vi "Dashboard Main.vi"() -> ()   [LabVIEW 2014]
uses:
  AutonModes.ctl
  <vilib>/event_ctls.llb/eventvkey.ctl
  <vilib>/Rock Robotics/WPI/Dashboard/WPI_DashboardLogging Global.vi
  <vilib>/Rock Robotics/Network Tables/SD Write String.vi
  <vilib>/Utility/config.llb/Write Key (String).vi
  <vilib>/Utility/config.llb/Write Key (I32).vi
  <vilib>/Utility/config.llb/NI_LVConfig.lvlib
panel:
  in  "TCP":refnum<k5>
  in  "Rec Mode":enum32{"Stop", "Record", "Playback"}(radio)
  in  "Vision":u16(ring) items=["Camera Off", "USB Camera SW", "USB Camera HW", "IP Camera"]
  out "Camera IP":string
  out "Image Message":string="Timeout in Camera Communications"
  in  "Dashboard Tab":T1(tab)
  in  "Camera Settings":T2={"Frame Rate"=30, "Compression"=30, "Size"=1} {"Frame Rate" scale=1.0..30.0; "Size" items=["640x480", "320x240", "160x120"]}
  out "MotorChart R":cluster{"Numeric":dbl, "Numeric":dbl}(graph)
  out "MotorChart L":T3(graph)
  out "MotorSliders R":cluster{"MotorSlide1":dbl, "MotorSlide2":dbl} {"MotorSlide2" scale=-1.0..1.0 scale format="%#_2e"; "MotorSlide1" scale=-1.0..1.0 scale format="%#_2e"}
  out "MotorSliders L":T4 {"MotorSlide4 2" scale=0.0..14.0 scale format="%#_2e"; "MotorSlide2" scale=-1.0..1.0 scale format="%#_2e"; "MotorSlide1" scale=-1.0..1.0 scale format="%#_2e"}
  out "Gyro":dbl(knob) scale=0.0..360.0
  out "JS1 Z":dbl(slide) scale=-1.0..1.0 scale format="%#_2e"
  out "JS1 Graph":cluster{"X":dbl, "Y":dbl}[](graph)
  out "JS1 Buttons":T5
  out "JS2 Z":dbl(slide) scale=-1.0..1.0 scale format="%#_2e"
  out "JS2 Graph":cluster{"X":dbl, "Y":dbl}[](graph)
  out "JS2 Buttons":T5
  out "Mode":T6(ring)=enum."Auto Disabled"
  in  "DB Camera Config":bool
  out "fps":dbl format="%#.1g"
  out "Mbps":dbl format="%#.1g"
  out "Mbps 2":bool
  in  "Auton Mode":T7
  in  "DB/String 9":string
  in  "DB/String 8":string
  in  "DB/String 7":string
  in  "DB/String 6":string
  in  "DB/String 5":string
  in  "DB/String 4":string
  in  "DB/String 3":string
  in  "DB/String 2":string
  in  "DB/String 1":string
  in  "DB/String 0":string
  in  "DB/Slider 0":dbl(slide) scale=0.0..5.0
  in  "DB/Slider 1":dbl(slide) scale=0.0..5.0
  in  "DB/Slider 2":dbl(slide) scale=0.0..5.0
  in  "DB/Slider 3":dbl(slide) scale=0.0..5.0
  out "DB/LED 3":bool
  out "DB/LED 2":bool
  out "DB/LED 1":bool
  out "DB/LED 0":bool
  in  "DB/Button 3":bool
  in  "DB/Button 2":bool
  in  "DB/Button 1":bool
  in  "DB/Button 0":bool caption="New Name"
  in  "Test Slider":dbl(slide) scale=0.0..100.0 scale format="%#_3g"
  in  "On/Off":bool caption="Solenoid"
  in  "Test Name":u16(ring) items=["Select the test to run...", "Example Test", "-------------------------------", "List of tests is built in robot code.", "Replace with your own automated tests."]
  in  "Test Tree":string(tree)
  in  "Motor":cluster{"Value":dbl, "Enable":bool} {"Value" scale=-1.0..1.0 scale format="%#_3g"}
  out "Progress":T8 {"Test Progress" scale=0.0..100.0}
  in  "Rev/Fwd":cluster{"Forward":bool, "Reverse":bool}
  in  "Test Ring":u16(ring) items=["Monochrome", "Color"]
  in  "Listbox":i32(listbox)
  out "Tree":string(tree)
  out "Camera Image":T9(plugin-control)
  out "Boolean":bool
  # "Left"
  # "Front"
  # "Right"
  # "Battery"
  # "This tab is a great place for autonomous settings and robot-specific values.\nPlace controls and indicators inside this tab and match name to\nDashboard Variables on robot. You can also delete this comment."
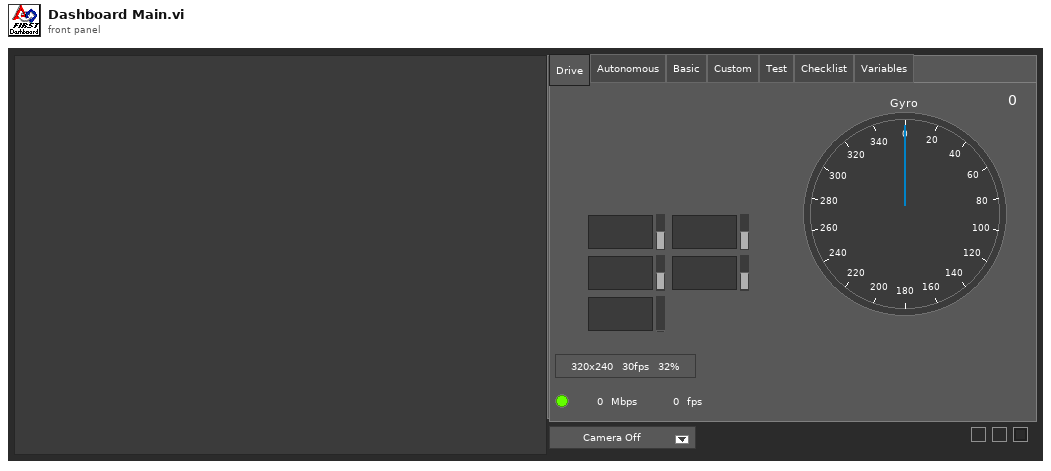
[diagram p1: front panel]
types:
  T1 = enum32{"Drive", "Autonomous", "Basic", "Custom", "Test", "Checklist", "Variables"}
  T2 = cluster{"Frame Rate":i32, "Compression":i32, "Size":u16}
  T3 = cluster{"Numeric":dbl, "Numeric":dbl, "Battery V":dbl}
  T4 = cluster{"MotorSlide1":dbl, "MotorSlide2":dbl, "MotorSlide4 2":dbl}
  T5 = cluster{bool, bool, bool, bool, bool, bool, bool, bool, bool, bool, bool, bool}
  T6 = enum8{"Tele-Op Disabled", "Tele-Op Enabled", "Auto Disabled", "Auto Enabled", "Test Disabled", "Test Enabled", "Disconnected", "No Code", "E-Stop"}
  T7 = typedef "AutonModes.ctl" = enum32{"Preset 1", "Preset 2", "Custom 1"}
  T8 = cluster{"Test Progress":u8, "Test Progress Text":string}
  T9 = typedef "IMAQ Image.ctl" = refnum<image>
  T10 = enum32{"Drive", "Basic", "Custom", "Test", "Checklist", "Variables"}
  T11 = typedef "Image Type" = u32
  T12 = cluster{"Camera Image":refnum<vi>, "Dashboard Tab":refnum<vi>, "Boolean":refnum<vi>, "Vision":refnum<vi>, "Rec Mode":refnum<vi>, "Test Slider":refnum<vi>, "On/Off ":refnum<vi>, "Test Ring":refnum<vi>, "Rev/Fwd":refnum<vi>, "Test Name":refnum<vi>, "Motor":refnum<vi>, "Progress":refnum<vi>, "CheckList":refnum<vi>, "Tree":refnum<vi>, "Test Tree":refnum<vi>}
  T13 = cluster{"Error Strings":string, "Disable Counts":cluster{u16, u16}, "Rail Faults":cluster{u16, u16, u16}, "Robot IP":string, "DB Mode":u8, "Event Info":cluster{"Name":string, "Type":u8, "Number":u16, "Replay":u8}, "Camera Addr":string}
  T14 = cluster{"Storage":cluster{"Disk Free":u64, "RAM Block":u32, "RAM free":u32}, "CPU Utilization":cluster{"CPU % ISR":sgl, "CPU % Time Crit":sgl, "CPU % Timed Str":sgl, "CPU % High":sgl, "CPU % Above":sgl, "CPU % Normal":sgl, "CPU % Low":sgl}, "CAN":cluster{"% Bus Utilization":sgl, "Bus Off Cnt":u32, "TX_FIFO Full Cnt":u32, "Receive Error Cnt":u8, "Transmit Error Cnt":u8}, "HID":cluster{"HID Outputs":u32, "Rumble Low":u16, "Rumble High":u16}[]}
  T15 = cluster{"Status bits":cluster{"Test Mode":bool, "Autonomous":bool, "Enabled":bool, "Code Start":bool, "Brownout":bool, "Reserved 2":bool, "Reserved 3":bool, "E-Stop":bool}, "Code Trace":cluster{"Disabled":bool, "TeleOp":bool, "Auto":bool, "Test":bool}, "Controller Type":enum16{"unknown", "cRIO", "roboRio"}, "Code?":enum16{"unknown", "noCode", "code"}, "Battery V":dbl}
  T16 = cluster{"Control Bits":cluster{"TestMode":bool, "Autonomous":bool, "Enabled":bool, "FMS Present":bool, bool, bool, bool, "E-Stop":bool}, "Team Station ":u8, "Countdown":sgl, "Joystick Values":cluster{"Axes":dbl[], "Buttons":bool[], "POVs":i16[]}[]}
  T17 = cluster{"Axes":dbl[], "Buttons":bool[], "POVs":i16[]}[]
  T18 = cluster{"Axes":dbl[], "Buttons":bool[], "POVs":i16[]}
  T19 = cluster{"Buttons[0]":bool, "Buttons[1]":bool, "Buttons[2]":bool, "Buttons[3]":bool, "Buttons[4]":bool, "Buttons[5]":bool, "Buttons[6]":bool, "Buttons[7]":bool, "Buttons[8]":bool, "Buttons[9]":bool, "Buttons[10]":bool, "Buttons[11]":bool}
  T20 = typedef "NI_LVConfig.lvlib/Config Data RefNum.ctl" = refnum<k1>
  T21 = cluster{"Operation":enum16{"Update", "Clear"}, "Color Box":u32}[]
  T22 = typedef "eventvkey.ctl" = enum16{"ASCII", "Enter", "Return", "Shift", "Ctrl", "Alt", "Cmd", "Opt", "Caps", "NumLock", "Clear", "Break", "Up", "Down", "Left", "Right", "Insert", "Delete", "Home", "End", "PageUp", "PageDown", "Escape", "Help", "Pause", "ScrollLock", "F1", "F2", "F3", "F4", "F5", "F6", "F7", "F8", "F9", "F10", "F11", "F12", "F13", "F14", "F15", "F16", "F17", "F18", "F19", "F20", "F21", "F22", "F23", "F24", "Play", "VolumeUp", "VolumeDown", "Mute", "Two Byte Char"}
  T23 = cluster{"Image Size":bool, "Image Type":bool, "Pixel Value":bool, "ROI Information":bool, "Zoom Factor":bool}
  T24 = enum8{"Enabled", "Disabled", "Disabled and Grayed Out"}
  T25 = cluster{"Operation":enum16{"Update", "Clear"}, "Color Box":u32}
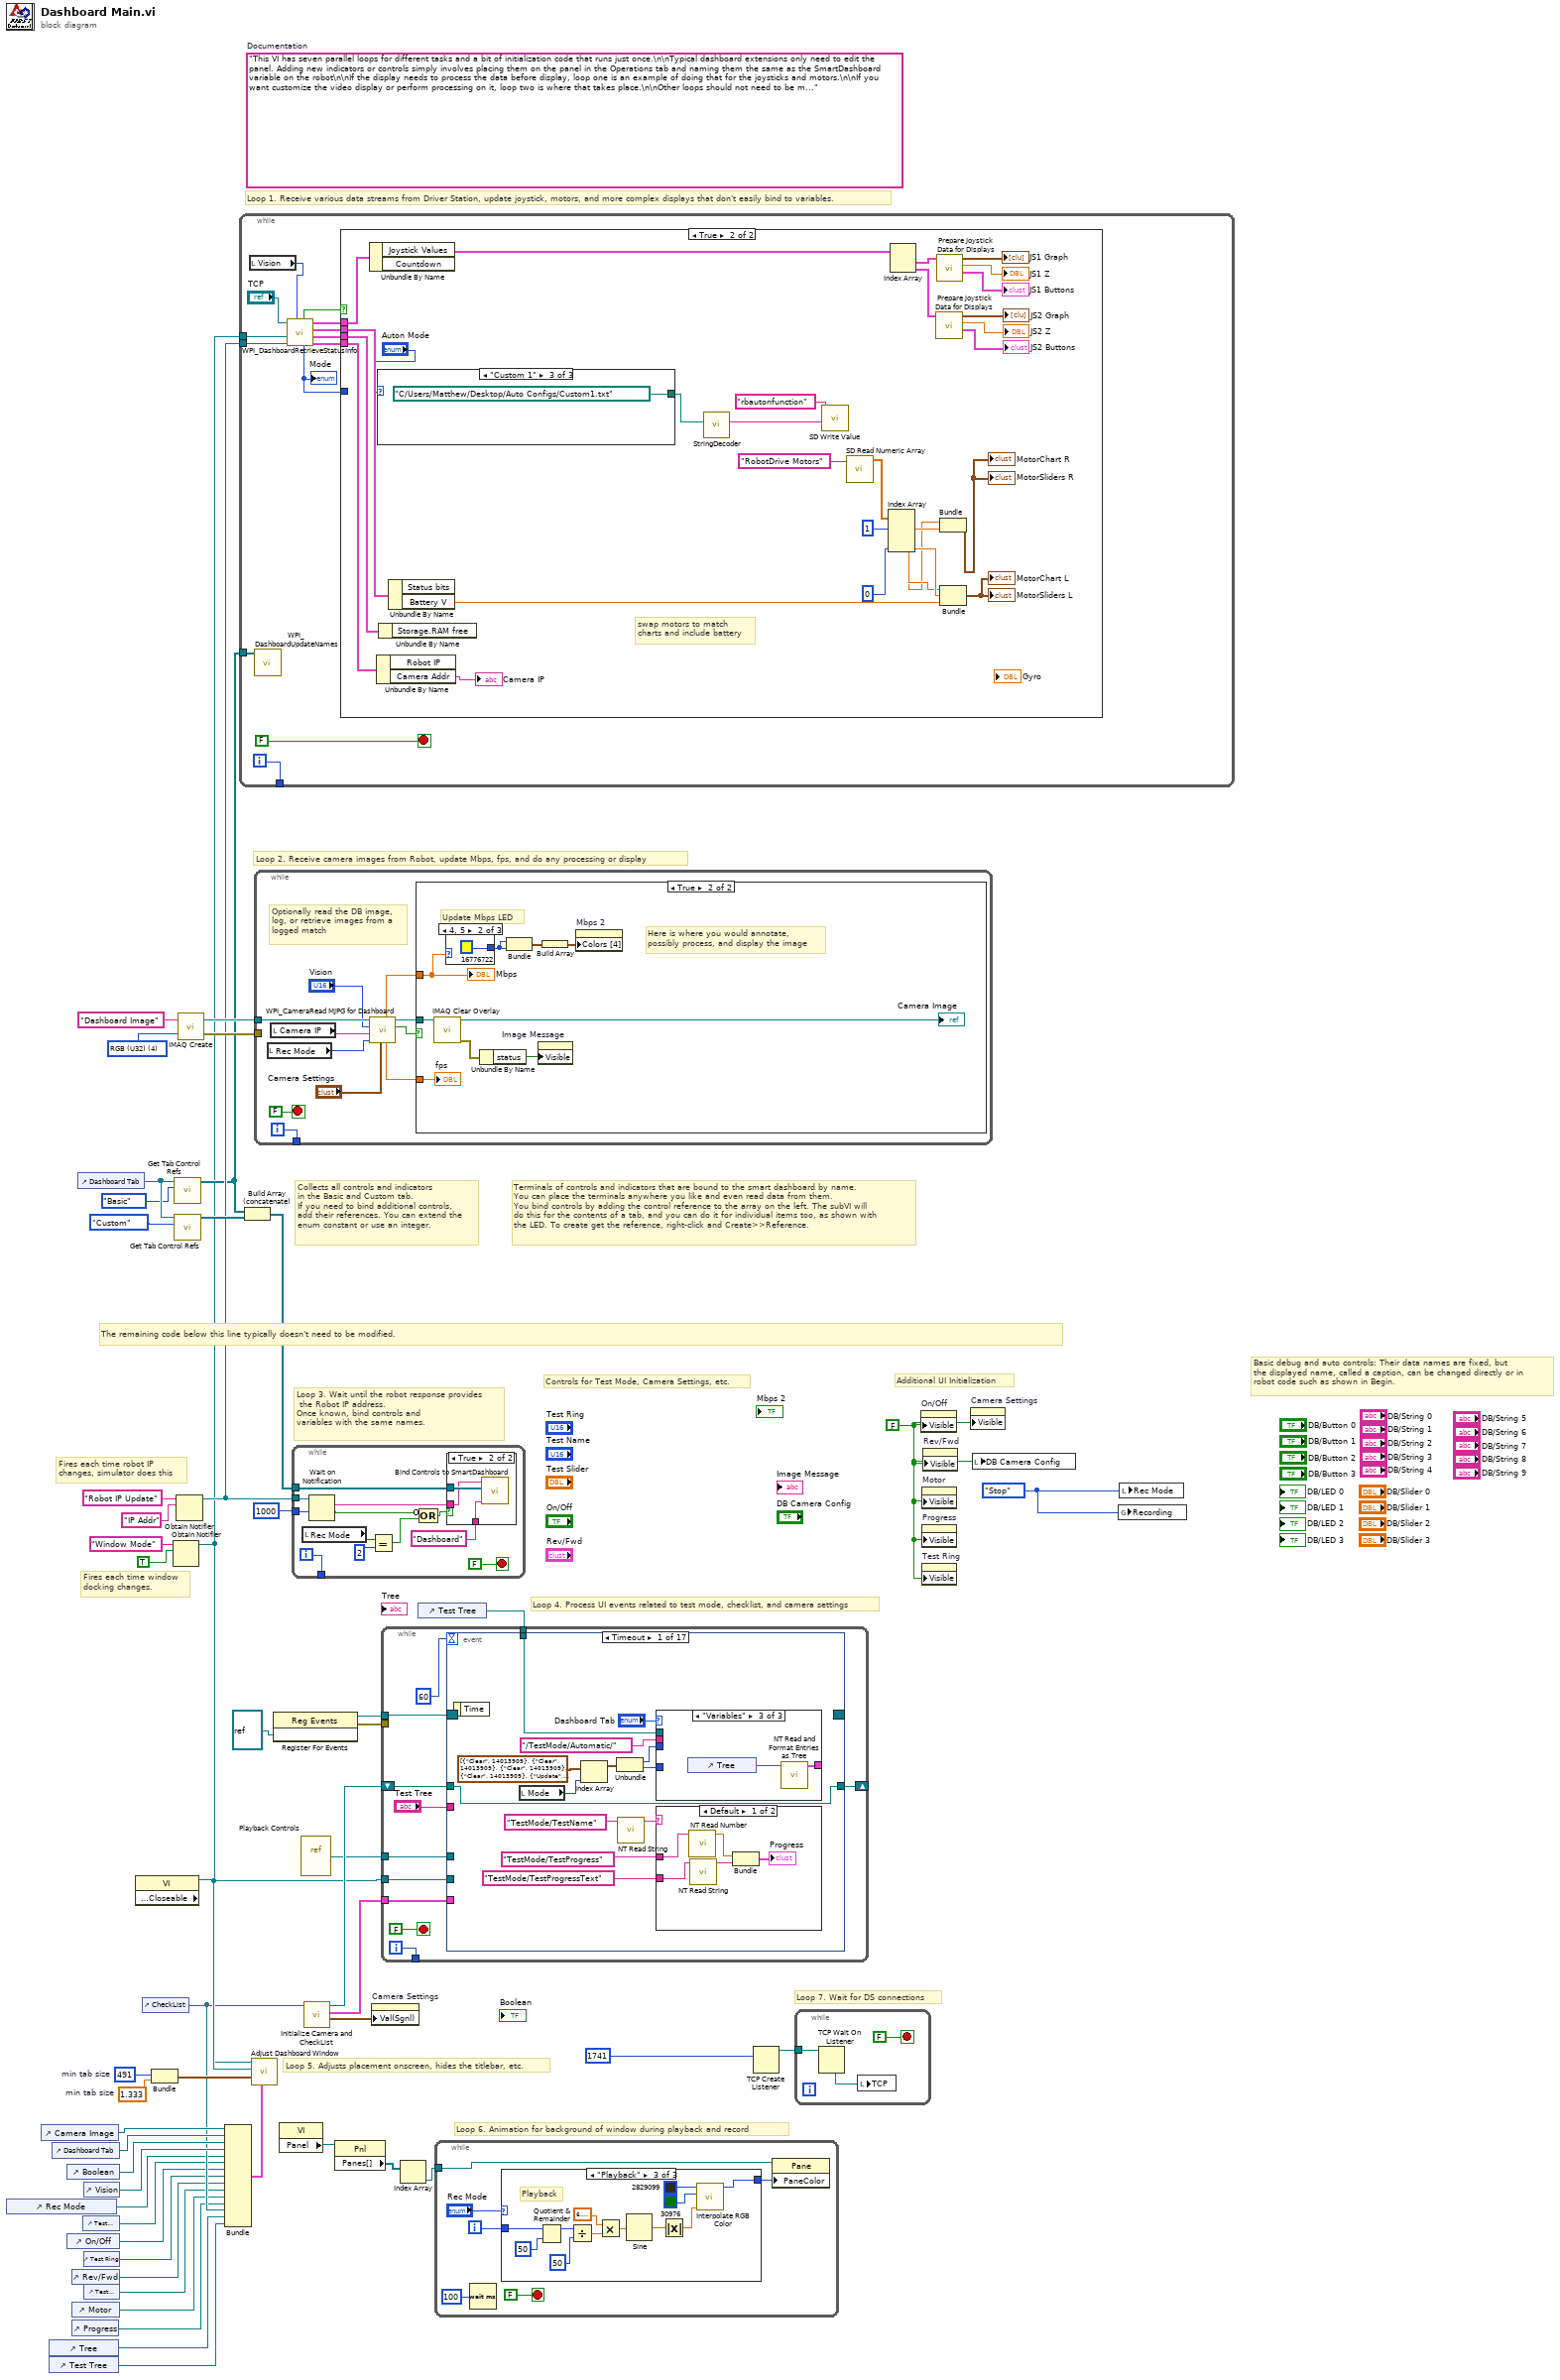
[diagram p0: block diagram]
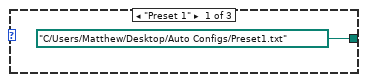
[diagram p3: hidden frame]
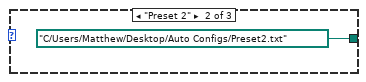
[diagram p4: hidden frame]
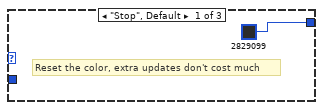
[diagram p5: hidden frame]
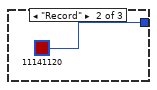
[diagram p6: hidden frame]
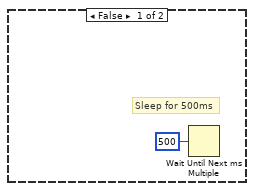
[diagram p8: hidden frame]
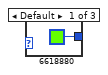
[diagram p9: hidden frame]
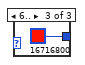
[diagram p10: hidden frame]
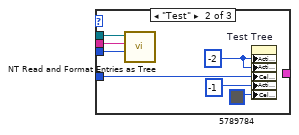
[diagram p12: hidden frame]
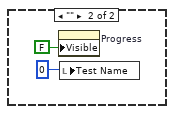
[diagram p13: hidden frame]
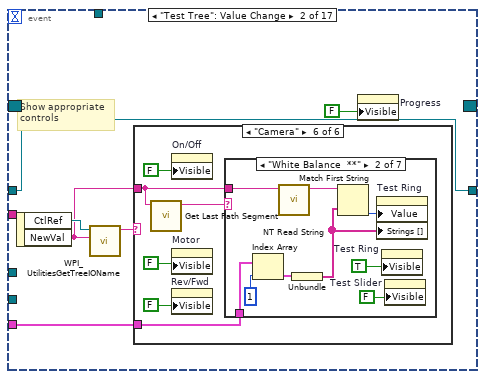
[diagram p14: hidden frame]
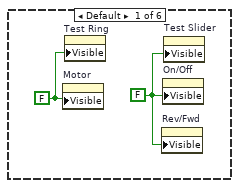
[diagram p15: hidden frame]
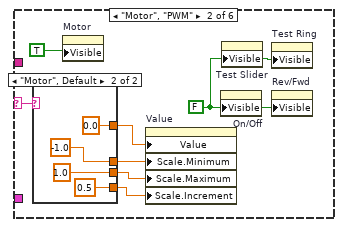
[diagram p16: hidden frame]
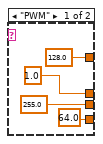
[diagram p17: hidden frame]
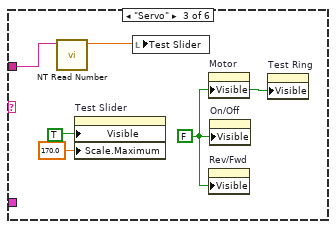
[diagram p18: hidden frame]
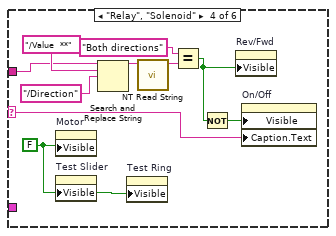
[diagram p19: hidden frame]
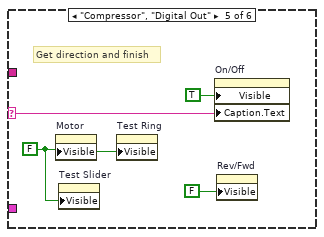
[diagram p20: hidden frame]
diagram:
  w24 = 491  # min tab size
  w23 = 1.333  # min tab size
  w32 = enum32{"Stop", "Record", "Playback"}."Stop" ("Rec Mode")
  w6 = FALSE ("Visible")
  (unwired) "This VI has seven parallel loops for different tasks and a bit of initialization code that runs just once.\n\nTypical dashboard extensions only need to edit the panel. Adding new indicators or controls simply involves placing them on the panel in the Operations tab and naming them the same as the SmartDashboard variable on the robot\n\nIf the display needs to process the data before display, loop one is an example of doing that for the joysticks and motors.\n\nIf you want customize the video display or perform processing on it, loop two is where that takes place.\n\nOther loops should not need to be modified. They are pretty standard, and document the task they perform."  # Documentation
  w52 = T11 4 items=["Grayscale (U8)", "Grayscale (I16)", "Grayscale (SGL)", "Complex (CSG)", "RGB (U32)", "HSL (U32)", "RGB (U64)"] ("Image Type")
  # "Loop 7. Wait for DS connections"
  # "Basic debug and auto controls: Their data names are fixed, but\nthe displayed name, called a caption, can be changed directly or in\nrobot code such as shown in Begin."
  # "Controls for Test Mode, Camera Settings, etc."
  # "Additional UI Initialization"
  # "Loop 6. Animation for background of window during playback and record"
  # "Fires each time robot IP\nchanges, simulator does this"
  # "Fires each time window\ndocking changes."
  # "Collects all controls and indicators\nin the Basic and Custom tab.\nIf you need to bind additional controls,\nadd their references. You can extend the\nenum constant or use an integer."
  # "The remaining code below this line typically doesn't need to be modified."
  # "Loop 4. Process UI events related to test mode, checklist, and camera settings"
  # "Terminals of controls and indicators that are bound to the smart dashboard by name.\nYou can place the terminals anywhere you like and even read data from them.\nYou bind controls by adding the control reference to the array on the left. The subVI will\ndo this for the contents of a tab, and you can do it for individual items too, as shown with\nthe LED. To create get the reference, right-click and Create>>Reference."
  # "Loop 3. Wait until the robot response provides\n the Robot IP address.\nOnce known, bind controls and\nvariables with the same names."
  # "Loop 5. Adjusts placement onscreen, hides the titlebar, etc."
  # "Loop 1. Receive various data streams from Driver Station, update joystick, motors, and more complex displays that don't easily bind to variables."
  # "Loop 2. Receive camera images from Robot, update Mbps, fps, and do any processing or display"
  n1 = control-ref of="Rec Mode"() -> (w12:refnum<vi>)
  n2 = control-ref of="Camera Image"() -> (w27:refnum<vi>)
  n3 = control-ref of="Tree"() -> (w16:refnum<vi>)
  n4 = control-ref of="Test Tree"() -> (w15:refnum<vi>)
  n5 = control-ref of="Dashboard Tab"() -> (w26:refnum<vi>)
  n6 = control-ref of="Boolean"() -> (w21:refnum<vi>)
  n7 = control-ref of="On/Off"() -> (w10:refnum<vi>)
  n8 = control-ref of="Progress"() -> (w7:refnum<vi>)
  n9 = control-ref of="Rev/Fwd"() -> (w8:refnum<vi>)
  n10 = control-ref of="Motor"() -> (w13:refnum<vi>)
  n11 = control-ref of="Dashboard Tab"() -> (w30:refnum<vi>)
  n12 = control-ref of="Test Slider"() -> (w11:refnum<vi>)
  n13 = control-ref of="Vision"() -> (w25:refnum<vi>)
  n14 = control-ref of="Test Ring"() -> (w9:refnum<vi>)
  n15 = control-ref of="Test Name"() -> (w14:refnum<vi>)
  n16 = property class="VI" props=["Front Panel.Closeable"]() -> (reference out=w31:refnum<vi>)  [unwired: 2 in, 2 out]
  n17 = control-ref of="CheckList"() -> (w17:refnum<vi>)
  n18 = Bundle("min tab size"=w24, "min tab size"=w23) -> (w22:cluster{"min tab size":i32, "min tab size":dbl})  [unwired: 1 in]
  n19 = Obtain Notifier(name (unnamed)="Window Mode", notification data type=TRUE) -> (notifier out=w3:refnum<notifier>)  [unwired: 2 in, 2 out]
  n20 = call <vilib>:"Get Tab Control Refs.vi"("Page Index"=T10."Basic" ("Dashboard Tab"), "TabControl in"=w30) -> ("ControlsOnPage"=w4:refnum<vi>[])  [unwired: 9 in]
  n21 = call <vilib>:"Get Tab Control Refs.vi"("Page Index"=T10."Custom" ("Dashboard Tab"), "TabControl in"=w30) -> ("ControlsOnPage"=w29:refnum<vi>[])  [unwired: 9 in]
  n22 = Obtain Notifier(name (unnamed)="Robot IP Update", notification data type="IP Addr" ("name (unnamed)")) -> (notifier out=w5:refnum<notifier>)  [unwired: 2 in, 2 out]
  n23 = call "IMAQ Create"("Image Name"="Dashboard Image", "Image Type"=w52) -> ("New Image"=w50:T9, "error out"=w49:errorcluster)  [unwired: 2 in, 1 out]
  n24 = Bundle("Camera Image"=w27, "Dashboard Tab"=w26, "Boolean"=w21, "Vision"=w25, "Rec Mode"=w12, "Test Slider"=w11, "On/Off"=w10, "Test Ring"=w9, "Rev/Fwd"=w8, "Test Name"=w14, "Motor"=w13, "Progress"=w7, "CheckList"=w17, "Tree"=w16, "Test Tree"=w15) -> (w18:T12)  [unwired: 1 in]
  n25 = while {
    tunnel: [w64] -> _
    tunnel: w5 -> [w58]
    tunnel: w4 -> [w57]
    tunnel: w3 -> [w53]
    i -> [w64]
    stop <- FALSE stop-if-true
    n26 = local read "Vision"() -> (w55:u16)
    n27 = call <vilib>:"WPI_DashboardUpdateNames.vi"("Controls on Tab"=w57) -> ()  [unwired: 11 in]
    n28 = call <vilib>:"WPI_DashboardRetrieveStatusInfo.vi"("Vision"=w55, "Binding Refnum"=w58, "Window Mode Notifier"=w53, "TCP Cnx"="TCP") -> ("Power and Errors"=w59:T13, "Robot Metrics"=w62:T14, "Status Info"=w63:T15, "Control Info"=w60:T16, "Robot Mode"=w56:T6, "Process?"=w61:bool)  [unwired: 2 in]
    "Mode" <- w56
    n29 = case shown="True" w61 {
      tunnel: w63 -> [_ w94]
      tunnel: w62 -> [_ w93]
      tunnel: w60 -> [_ w92]
      tunnel: w59 -> [_ w91]
      tunnel: w56 -> [_ _]
      frame False {
      }
      frame True {
        # "swap motors to match\ncharts and include battery"
        n30 = Unbundle By Name(w92) -> ("Joystick Values"=w79:T17)  [unwired: 1 out]
        n31 = Unbundle By Name(w91) -> ("Camera Addr"=→"Camera IP":string)  [unwired: 1 out]
        n32 = case shown="\"Custom 1\"" "Auton Mode" {
          tunnel: [path "C:/Users/Matthew/Desktop/Auto Configs/Preset1.txt" ("Path") path "C:/Users/Matthew/Desktop/Auto Configs/Preset2.txt" ("Path") path "C:/Users/Matthew/Desktop/Auto Configs/Custom1.txt" ("Path")] -> w68
          frame "Preset 1" {
          }
          frame "Preset 2" {
          }
          frame "Custom 1" {
          }
        }
        n33 = Unbundle By Name(w93) -> ()  [unwired: 1 out]
        n34 = Unbundle By Name(w94) -> ("Battery V"=w80:dbl)  [unwired: 1 out]
        n35 = call "StringDecoder.vi"("Auto Config File"=w68) -> ("RobotDataString"=w67:string)  [unwired: 10 in]
        n36 = call-poly <vilib>:"SD Write Value.vi"("String"=w67, "Name"="rbautonfunction") -> ()  [unwired: 8 in, 2 out]
        n37 = call <vilib>:"SD Read Numeric Array.vi"("Name"="RobotDrive Motors") -> ("Numeric Array"=w82:dbl[])  [unwired: 8 in, 2 out]
        n38 = Index Array(array=w82, index #1=1, index #4=0) -> (element #1=w86:dbl, element #2=w87:dbl, element #3=w85:dbl, element #4=w90:dbl)  [unwired: 2 in]
        n39 = Index Array(array=w79) -> (element #1=w78:T18, element #2=w73:T18)  [unwired: 2 in]
        n40 = call "Prepare Joystick Data for Displays.vi"("Joystick Values"=w73) -> ("Buttons"=→"JS2 Buttons":T19, "Z Axis"=→"JS2 Z":dbl, "Cartesian Data"=→"JS2 Graph":cluster{"X axis":dbl, "X axis":dbl}[])  [unwired: 8 in]
        n41 = call "Prepare Joystick Data for Displays.vi"("Joystick Values"=w78) -> ("Buttons"=→"JS1 Buttons":T19, "Z Axis"=→"JS1 Z":dbl, "Cartesian Data"=→"JS1 Graph":cluster{"X axis":dbl, "X axis":dbl}[])  [unwired: 8 in]
        n42 = Bundle("Numeric"=w85, "Numeric"=w86) -> (→"MotorChart R" →"MotorSliders R":cluster{"Numeric":dbl, "Numeric":dbl})  [unwired: 1 in]
        n43 = Bundle("Numeric"=w87, "Numeric"=w90, "Battery V"=w80) -> (→"MotorChart L" →"MotorSliders L":T3)  [unwired: 1 in]
      }
    }
  }
  n44 = Build Array (concatenate)(w4, w29) -> (w28:refnum<vi>[])
  n45 = call "Adjust Dashboard Window.vi"("Sizing Refnums"=w18, "Size Constraints"=w22, "VI"=w31, "Notifier in"=w3) -> ()  [unwired: 8 in]
  n46 = while {
    tunnel: w50 -> [w106]
    tunnel: w49 -> [_]
    tunnel: [w107] -> _
    i -> [w107]
    stop <- FALSE stop-if-true
    # "Optionally read the DB image,\nlog, or retrieve images from a\nlogged match"
    n47 = local read "Rec Mode"() -> (w100:enum32{"Stop", "Record", "Playback"})
    n48 = local read "Camera IP"() -> (w98:string)
    n49 = call <vilib>:"WPI_CameraRead MJPG for Dashboard.vi"("Camera Settings"="Camera Settings", "Rec Mode"=w100, "Camera IP"=w98, "Camera Mode"="Vision", "Refnum in"=w106) -> ("Active"=w104:bool, "Refnum out"=w105:T9, "FPS"=w103:dbl, "Bandwidth (Mbps)"=w102:dbl)  [unwired: 3 in]
    n50 = case shown="True" w104 {
      tunnel: w105 -> [_ w113]
      tunnel: w102 -> [_ w112]
      tunnel: w103 -> [_ w110]
      frame False {
        # "Sleep for 500ms"
        n51 = Wait Until Next ms Multiple(millisecond multiple=u32 500) -> ()  [unwired: 1 out]
      }
      frame True {
        # "Here is where you would annotate,\npossibly process, and display the image"
        # "Update Mbps LED"
        n52 = call "IMAQ Clear Overlay"("Image"=w113) -> ("error out"=w117:errorcluster, "Image Out"=→"Camera Image":T9)  [unwired: 2 in, 7 out]
        n53 = case shown="4, 5" w112 {
          tunnel: [u32 6618880 ("Color Box") u32 16776722 ("Color Box") u32 16716800 ("Color Box")] -> w114
          frame Default {
          }
          frame 4, 5 {
          }
          frame 6.. {
          }
        }
        n54 = Unbundle By Name(w117) -> ("status"=w118:bool)
        n55 = Bundle("Color Box"=w114, "Color Box"=w114) -> (w116:cluster{"Color Box":u32, "Color Box":u32})  [unwired: 1 out]
        n56 = property on="Image Message" class="Str"("Visible"=w118) -> ()  [unwired: 2 in, 2 out]
        n57 = Build Array(w116) -> (w115:cluster{"Color Box":u32, "Color Box":u32}[])
        n58 = property on="Mbps 2" class="Bool (strict)"("Colors [4]"=w115) -> ()  [unwired: 2 in, 2 out]
        "Mbps" <- w112
        "fps" <- w110
      }
    }
  }
  n59 = register-events(refnum<vi> refnum) -> (reference out=w36:refnum<event-registration>, error out=w35:errorcluster)  [unwired: 2 in]
  n60 = property class="VI"() -> ("Panel"=w39:refnum<vi>)  [unwired: 2 in, 2 out]
  n61 = while {
    tunnel: w28 -> [w133]
    tunnel: w5 -> [w131]
    tunnel: [w129] -> _
    tunnel: u32 1000 ("milliseconds to wait") -> [w128]
    i -> [w129]
    stop <- FALSE stop-if-true
    n62 = local read "Rec Mode"() -> (w124:enum32{"Stop", "Record", "Playback"})
    n63 = Wait on Notification(notifier=w131, timeout in ms (-1)=w128) -> (notification=w130:string, timed out?=w126:bool)  [unwired: 2 in, 2 out]
    n64 = Equal?(x=w124, y=u16 2 ("Rec Mode")) -> (x = y?=w125:bool)
    n65 = Compound Arithmetic op=OR(invert w126, w125) -> (w127:bool)
    n66 = case shown="True" w127 {
      tunnel: w133 -> [_ w136]
      tunnel: w130 -> [_ w135]
      tunnel: "Dashboard" -> [_ w134]
      frame False {
      }
      frame True {
        n67 = call <vilib>:"Bind Controls to SmartDashboard.vi"("Client Name"=w134, "Bound Control Refs"=w136, "Server IP Address"=w135) -> ()  [unwired: 9 in]
      }
    }
  }
  n68 = vi-ref "Playback Controls.vi"() -> (w37:refnum<vi>)
  n69 = call "Initialize Camera and CheckList.vi"("ListBox in"=w17) -> ("Cluster"=w43:cluster{"value":i32, "value":i32, "index":i32}, "Array"=w44:cluster{string[]}[], "File Refnum"=w42:T20)  [unwired: 8 in]
  n70 = property class="Pnl"(reference=w39) -> ("Panes[]"=w40:refnum<vi>[])  [unwired: 1 in, 2 out]
  n71 = property on="Camera Settings" class="Clust (strict)"("Val(Sgnl)"=w43) -> ()  [unwired: 2 in, 2 out]
  n72 = Index Array(array=w40) -> (element=w38:refnum<vi>)  [unwired: 1 in]
  n73 = control-ref of="Test Tree"() -> (w41:refnum<vi>)
  n74 = while {
    tunnel: w44 -> [w144]
    shift-right: [w143] -> _
    shift-left: w42 -> [w142]
    tunnel: [w141] -> _
    tunnel: w41 -> [w140]
    tunnel: w37 -> [w139]
    tunnel: w36 -> [w138]
    tunnel: w35 -> [_]
    tunnel: w31 -> [w137]
    i -> [w141]
    stop <- FALSE stop-if-true
    n75 = event shown="[0] Timeout" {
      selector: w138 -> [_ _ _ _ _ _ _ _ _ _ _ _ _ _ _ _ _]
      dyn-events: [_ _ _ _ _ _ _ _ _ _ _ _ _ w382 _ _ _] -> _
      timeout: u32 60 ("milliseconds to wait") -> [_ _ _ _ _ _ _ _ _ _ _ _ _ _ _ _ _]
      tunnel: w140 -> [w156 _ _ _ _ _ _ _ _ _ _ _ _ _ _ _ _]
      tunnel: "Test Tree" -> [_ _ _ _ _ _ _ _ w351 w359 w361 w365 w373 _ _ _ _]
      tunnel: w144 -> [_ w178 _ _ _ _ w315 w345 _ _ _ _ _ _ _ _ _]
      tunnel: [w152 w177 w276 w281 w289 w301 w314 w338 w350 w357 w360 w364 w372 w384 w398 w399 w409] -> w143
      tunnel: w142 -> [w152 w177 w276 w281 w289 w301 w313 w338 w350 w357 w360 w364 w372 w384 w398 w399 w409]
      tunnel: w139 -> [_ _ _ _ _ _ _ _ _ _ _ _ _ w385 _ w402 _]
      tunnel: w137 -> [_ _ _ _ _ _ _ _ _ _ _ _ _ w380 _ _ _]
      event Timeout {
        n76 = event-data() -> ()  [unwired: 1 in, 1 out]
        n77 = local read "Mode"() -> (w155:T6)
        n78 = Index Array(array=T21 [{"Operation"=enum."Clear", "Color Box"=14013909}, {"Operation"=enum."Clear", "Color Box"=14013909}, {"Operation"=enum."Clear", "Color Box"=14013909}, {"Operation"=enum."Clear", "Color Box"=14013909}, {"Operation"=enum."Update", "Color Box"=14013909}, {"Operation"=enum."Update", "Color Box"=16777215}, {"Operation"=enum."Clear", "Color Box"=14013909}, {"Operation"=enum."Clear", "Color Box"=14013909}, {"Operation"=enum."Clear", "Color Box"=14013909}], index=w155) -> (element=w150:T25)
        n79 = Unbundle(w150) -> ("Operation"=w149:enum16{"Update", "Clear"}, "Color Box"=w148:u32)
        n80 = call <vilib>:"NT Read String.vi"("Name"="TestMode/TestName") -> ("String"=w159:string)  [unwired: 9 in, 1 out]
        n81 = case shown="\"Variables\"" "Dashboard Tab" {
          tunnel: w156 -> [_ w167 _]
          tunnel: "/TestMode/Automatic/" ("Name Pattern") -> [_ w166 _]
          tunnel: w149 -> [_ w165 _]
          tunnel: [_ _ w169] -> _
          tunnel: w148 -> [_ w161 _]
          frame "Custom", Default {
          }
          frame "Test" {
            w164 = -2 ("Active Item:Row Number")
            n82 = call <vilib>:"NT Read and Format Entries as Tree.vi"("Operation"=w165, "Name Pattern"=w166, "Tree Refnum"=w167) -> ()  [unwired: 7 in, 2 out]
            n83 = property on="Test Tree" class="Tree (strict)"("Active Item Row Number"=w164, "ActiveColNum"=w164, "CellBG"=w161, "Active Item Row Number"=-1 ("Active Item:Row Number"), "CellBG"=u32 5789784 ("Color Box")) -> ()  [unwired: 2 in, 2 out]
          }
          frame "Variables" {
            n84 = control-ref of="Tree"() -> (w168:refnum<vi>)
            n85 = call <vilib>:"NT Read and Format Entries as Tree.vi"("Tree Refnum"=w168) -> ("Formatted Strings"=w169:cluster{"Name":string, "Value":string}[])  [unwired: 9 in, 1 out]
          }
        }
        n86 = case shown="Default" w159 {
          tunnel: "TestMode/TestProgress" ("Name") -> [w171 _]
          tunnel: "TestMode/TestProgressText" ("Name") -> [w170 _]
          frame Default {
            n87 = call <vilib>:"NT Read Number.vi"("Name"=w171) -> ("Numeric"=w172:dbl)  [unwired: 9 in, 1 out]
            n88 = call <vilib>:"NT Read String.vi"("Name"=w170) -> ("String"=w173:string)  [unwired: 9 in, 1 out]
            n89 = Bundle("Numeric"=w172, "String"=w173) -> (→"Progress":cluster{"Numeric":dbl, "String":string})  [unwired: 1 in]
          }
          frame "" {
            n90 = property on="Progress" class="Clust (strict)"("Visible"=FALSE) -> ()  [unwired: 2 in, 2 out]
            n91 = local write "Test Name"(u16 0) -> ()
          }
        }
      }
      event "Test Tree": Value Change {
        # "Show appropriate\ncontrols"
        n92 = event-data() -> ("CtlRef"=w181:refnum<vi>, "NewVal"=w179:string)  [unwired: 1 in]
        n93 = call <vilib>:"WPI_UtilitiesGetTreeIOName.vi"("NewVal"=w179, "TreeControl in"=w181) -> ("I/O Name"=w182:string)  [unwired: 9 in]
        n94 = case shown="\"Camera\"" w182 {
          selector: w182 -> [_ w189 _ w207 w216 _]
          tunnel: w179 -> [_ _ w204 w206 _ w223]
          tunnel: w178 -> [_ _ _ _ _ w222]
          frame Default {
            w184 = FALSE ("Visible")
            w183 = FALSE ("Visible")
            n95 = property on="Motor" class="Clust (strict)"("Visible"=w183) -> ()  [unwired: 2 in, 2 out]
            n96 = property on="Test Ring" class="Ring (strict)"("Visible"=w183) -> ()  [unwired: 2 in, 2 out]
            n97 = property on="Rev/Fwd" class="Clust (strict)"("Visible"=w184) -> ()  [unwired: 2 in, 2 out]
            n98 = property on="On/Off" class="Bool (strict)"("Visible"=w184) -> ()  [unwired: 2 in, 2 out]
            n99 = property on="Test Slider" class="Slide (strict)"("Visible"=w184) -> ()  [unwired: 2 in, 2 out]
          }
          frame "Motor", "PWM" {
            w190 = FALSE ("Visible")
            n100 = case shown="\"Motor\", Default" w189 {
              tunnel: [1.0 ("Value") -1.0 ("Value")] -> w188
              tunnel: [255.0 ("Value") 1.0 ("Value")] -> w187
              tunnel: [128.0 ("Value") 0.0 ("Value")] -> w186
              tunnel: [64.0 ("Value") 0.5 ("Value")] -> w185
              frame "PWM" {
              }
              frame "Motor", Default {
              }
            }
            n101 = property on="Motor" class="Clust (strict)"("Visible"=TRUE) -> ()  [unwired: 2 in, 2 out]
            n102 = property on="Value" class="Slide (strict)"("Value"=w186, "Scale.Minimum"=w188, "Scale.Maximum"=w187, "Scale.Increment"=w185) -> ()  [unwired: 2 in, 2 out]
            n103 = property on="On/Off" class="Bool (strict)"("Visible"=w190) -> ()  [unwired: 2 in, 2 out]
            n104 = property on="Test Slider" class="Slide (strict)"("Visible"=w190) -> ()  [unwired: 2 in, 2 out]
            n105 = property on="Test Ring" class="Ring (strict)"("Visible"=w190) -> ()  [unwired: 2 in, 2 out]
            n106 = property on="Rev/Fwd" class="Clust (strict)"("Visible"=w190) -> ()  [unwired: 2 in, 2 out]
          }
          frame "Servo" {
            w202 = FALSE ("Visible")
            n107 = call <vilib>:"NT Read Number.vi"("Name"=w204) -> ("Numeric"=w203:dbl)  [unwired: 9 in, 1 out]
            n108 = property on="Test Slider" class="Slide (strict)"("Visible"=TRUE, "Scale.Maximum"=170.0 ("Scale.Range:Maximum")) -> ()  [unwired: 2 in, 2 out]
            n109 = local write "Test Slider"(w203) -> ()
            n110 = property on="Motor" class="Clust (strict)"("Visible"=w202) -> ()  [unwired: 2 in, 2 out]
            n111 = property on="Rev/Fwd" class="Clust (strict)"("Visible"=w202) -> ()  [unwired: 2 in, 2 out]
            n112 = property on="On/Off" class="Bool (strict)"("Visible"=w202) -> ()  [unwired: 2 in, 2 out]
            n113 = property on="Test Ring" class="Ring (strict)"("Visible"=w202) -> ()  [unwired: 2 in, 2 out]
          }
          frame "Relay", "Solenoid" {
            w205 = FALSE ("Visible")
            n114 = property on="Motor" class="Clust (strict)"("Visible"=w205) -> ()  [unwired: 2 in, 2 out]
            n115 = property on="Test Slider" class="Slide (strict)"("Visible"=w205) -> ()  [unwired: 2 in, 2 out]
            n116 = Search and Replace String(input string=w206, search string="/Value  **", replace string="/Direction") -> (result string=w212:string)  [unwired: 5 in, 3 out]
            n117 = property on="Test Ring" class="Ring (strict)"("Visible"=w205) -> ()  [unwired: 2 in, 2 out]
            n118 = call <vilib>:"NT Read String.vi"("Name"=w212) -> ("String"=w210:string)  [unwired: 9 in, 1 out]
            n119 = Equal?(x="Both directions", y=w210) -> (x = y?=w208:bool)
            n120 = Not(x=w208) -> (.not. x?=w209:bool)
            n121 = property on="Rev/Fwd" class="Clust (strict)"("Visible"=w208) -> ()  [unwired: 2 in, 2 out]
            n122 = property on="On/Off" class="Bool (strict)"("Visible"=w209, "Caption.Text"=w207) -> ()  [unwired: 2 in, 2 out]
          }
          frame "Compressor", "Digital Out" {
            w215 = FALSE ("Visible")
            # "Get direction and finish"
            n123 = property on="Motor" class="Clust (strict)"("Visible"=w215) -> ()  [unwired: 2 in, 2 out]
            n124 = property on="Test Slider" class="Slide (strict)"("Visible"=w215) -> ()  [unwired: 2 in, 2 out]
            n125 = property on="Test Ring" class="Ring (strict)"("Visible"=w215) -> ()  [unwired: 2 in, 2 out]
            n126 = property on="On/Off" class="Bool (strict)"("Visible"=TRUE, "Caption.Text"=w216) -> ()  [unwired: 2 in, 2 out]
            n127 = property on="Rev/Fwd" class="Clust (strict)"("Visible"=FALSE) -> ()  [unwired: 2 in, 2 out]
          }
          frame "Camera" {
            n128 = call <vilib>:"Get Last Path Segment.vi"("String in"=w223) -> ("String out"=w224:string)  [unwired: 10 in]
            n129 = property on="On/Off" class="Bool (strict)"("Visible"=FALSE) -> ()  [unwired: 2 in, 2 out]
            n130 = property on="Motor" class="Clust (strict)"("Visible"=FALSE) -> ()  [unwired: 2 in, 2 out]
            n131 = property on="Rev/Fwd" class="Clust (strict)"("Visible"=FALSE) -> ()  [unwired: 2 in, 2 out]
            n132 = case shown="\"White Balance  **\"" w224 {
              tunnel: w223 -> [w230 w239 w248 w257 w266 _ w272]
              tunnel: w222 -> [w228 w236 w245 w254 w263 _ _]
              frame "Size  **" {
                n133 = Index Array(array=w228) -> (element=w227:cluster{string[]})  [unwired: 1 in]
                n134 = call <vilib>:"NT Read String.vi"("Name"=w230) -> ("String"=w229:string)  [unwired: 9 in, 1 out]
                n135 = Unbundle(w227) -> (w225:string[])
                n136 = Match First String(2:w225, 3:w229) -> (0:w226:i32)  [unwired: 1 out]
                n137 = property on="Test Ring" class="Ring (strict)"("Value"=w226, "Strings []"=w225) -> ()  [unwired: 2 in, 2 out]
                n138 = property on="Test Ring" class="Ring (strict)"("Visible"=TRUE) -> ()  [unwired: 2 in, 2 out]
                n139 = property on="Test Slider" class="Slide (strict)"("Visible"=FALSE) -> ()  [unwired: 2 in, 2 out]
              }
              frame "White Balance  **" {
                n140 = Index Array(array=w236, index=1) -> (element=w237:cluster{string[]})
                n141 = call <vilib>:"NT Read String.vi"("Name"=w239) -> ("String"=w238:string)  [unwired: 9 in, 1 out]
                n142 = Unbundle(w237) -> (w234:string[])
                n143 = Match First String(2:w234, 3:w238) -> (0:w233:i32)  [unwired: 1 out]
                n144 = property on="Test Ring" class="Ring (strict)"("Value"=w233, "Strings []"=w234) -> ()  [unwired: 2 in, 2 out]
                n145 = property on="Test Ring" class="Ring (strict)"("Visible"=TRUE) -> ()  [unwired: 2 in, 2 out]
                n146 = property on="Test Slider" class="Slide (strict)"("Visible"=FALSE) -> ()  [unwired: 2 in, 2 out]
              }
              frame "Exposure  **" {
                n147 = Index Array(array=w245, index=2) -> (element=w246:cluster{string[]})
                n148 = call <vilib>:"NT Read String.vi"("Name"=w248) -> ("String"=w247:string)  [unwired: 9 in, 1 out]
                n149 = Unbundle(w246) -> (w242:string[])
                n150 = Match First String(2:w242, 3:w247) -> (0:w243:i32)  [unwired: 1 out]
                n151 = property on="Test Ring" class="Ring (strict)"("Value"=w243, "Strings []"=w242) -> ()  [unwired: 2 in, 2 out]
                n152 = property on="Test Ring" class="Ring (strict)"("Visible"=TRUE) -> ()  [unwired: 2 in, 2 out]
                n153 = property on="Test Slider" class="Slide (strict)"("Visible"=FALSE) -> ()  [unwired: 2 in, 2 out]
              }
              frame "Exposure Priority  **" {
                n154 = Index Array(array=w254, index=3) -> (element=w255:cluster{string[]})
                n155 = call <vilib>:"NT Read String.vi"("Name"=w257) -> ("String"=w256:string)  [unwired: 9 in, 1 out]
                n156 = Unbundle(w255) -> (w251:string[])
                n157 = Match First String(2:w251, 3:w256) -> (0:w252:i32)  [unwired: 1 out]
                n158 = property on="Test Ring" class="Ring (strict)"("Value"=w252, "Strings []"=w251) -> ()  [unwired: 2 in, 2 out]
                n159 = property on="Test Ring" class="Ring (strict)"("Visible"=TRUE) -> ()  [unwired: 2 in, 2 out]
                n160 = property on="Test Slider" class="Slide (strict)"("Visible"=FALSE) -> ()  [unwired: 2 in, 2 out]
              }
              frame "Color Enable  **" {
                n161 = Index Array(array=w263, index=4) -> (element=w264:cluster{string[]})
                n162 = call <vilib>:"NT Read String.vi"("Name"=w266) -> ("String"=w265:string)  [unwired: 9 in, 1 out]
                n163 = Unbundle(w264) -> (w260:string[])
                n164 = Match First String(2:w260, 3:w265) -> (0:w261:i32)  [unwired: 1 out]
                n165 = property on="Test Ring" class="Ring (strict)"("Value"=w261, "Strings []"=w260) -> ()  [unwired: 2 in, 2 out]
                n166 = property on="Test Ring" class="Ring (strict)"("Visible"=TRUE) -> ()  [unwired: 2 in, 2 out]
                n167 = property on="Test Slider" class="Slide (strict)"("Visible"=FALSE) -> ()  [unwired: 2 in, 2 out]
              }
              frame Default {
                n168 = property on="Test Ring" class="Ring (strict)"("Visible"=FALSE) -> ()  [unwired: 2 in, 2 out]
                n169 = property on="Test Slider" class="Slide (strict)"("Visible"=FALSE) -> ()  [unwired: 2 in, 2 out]
              }
              frame "Brightness  **", "Color Level  **", "Compression  **", "FPS  **", "Sharpness  **" {
                n170 = call <vilib>:"NT Read Number.vi"("Name"=w272) -> ("Numeric"=w271:dbl)  [unwired: 9 in, 1 out]
                n171 = local write "Test Slider"(w271) -> ()
                n172 = property on="Test Slider" class="Slide (strict)"("Visible"=TRUE, "Scale.Maximum"=100.0 ("Scale.Range:Maximum")) -> ()  [unwired: 2 in, 2 out]
                n173 = property on="Test Ring" class="Ring (strict)"("Visible"=FALSE) -> ()  [unwired: 2 in, 2 out]
              }
            }
          }
        }
        n174 = property on="Progress" class="Clust (strict)"("Visible"=FALSE) -> ()  [unwired: 2 in, 2 out]
      }
      event "Test Name": Mouse Enter {
        # "Populate the ring with the list of tests"
        n175 = event-data() -> ()  [unwired: 1 in, 1 out]
        n176 = call <vilib>:"NT Read String Array.vi"("Name"="TestMode/TestList") -> ("String Array"=w280:string[])  [unwired: 9 in, 1 out]
        n177 = Build Array (concatenate)("Select the test to run...", w280) -> (w279:string[])
        n178 = property on="Test Name" class="Ring (strict)"("Strings []"=w279) -> ()  [unwired: 2 in, 2 out]
      }
      event "Test Name": Value Change {
        w282 = FALSE ("Visible")
        # "Tell the robot the test name to run"
        n179 = event-data() -> ("NewVal"=w286:u16)  [unwired: 1 in]
        n180 = property on="Test Name" class="Ring (strict)"() -> ("Strings []"=w287:string[])  [unwired: 2 in, 2 out]
        n181 = local write "Progress"(T8 {"Test Progress"=0, "Test Progress Text"=""} ("Progress")) -> ()
        n182 = Index Array(array=w287, index=w286) -> (element=w285:string)
        n183 = call <vilib>:"NT Write String.vi"("String"=w285, "Name"="TestMode/TestName") -> ()  [unwired: 9 in, 1 out]
        n184 = property on="Progress" class="Clust (strict)"("Visible"=TRUE) -> ()  [unwired: 2 in, 2 out]
        n185 = property on="Motor" class="Clust (strict)"("Visible"=w282) -> ()  [unwired: 2 in, 2 out]
        n186 = property on="Test Slider" class="Slide (strict)"("Visible"=w282) -> ()  [unwired: 2 in, 2 out]
        n187 = property on="On/Off" class="Bool (strict)"("Visible"=w282) -> ()  [unwired: 2 in, 2 out]
        n188 = property on="Rev/Fwd" class="Clust (strict)"("Visible"=w282) -> ()  [unwired: 2 in, 2 out]
        n189 = property on="Test Ring" class="Ring (strict)"("Visible"=w282) -> ()  [unwired: 2 in, 2 out]
      }
      event "Listbox": Double Click {
        # "Shift clears all"
        # "Update symbols on the listbox"
        n190 = event-data() -> ("PlatMods.Shift"=w290:bool, "Row"=w292:i32)  [unwired: 1 in]
        n191 = case shown="True" w290 {
          tunnel: w292 -> [w296 _]
          tunnel: 1 -> [w295 _]
          frame False {
            n192 = property on="Listbox" class="LstBox (strict)"() -> ("Item Symbols"=w294:i32[])  [unwired: 2 in, 2 out]
            n193 = Replace Array Subset(array=w294, new element=w295, index=w296) -> (w293:i32[])
            n194 = property on="Listbox" class="LstBox (strict)"("Item Symbols"=w293) -> ()  [unwired: 2 in, 2 out]
          }
          frame True {
            w297 = 0 ("Top Row")
            n195 = property on="Listbox" class="LstBox (strict)"() -> ("Number of Rows"=w299:u32)  [unwired: 2 in, 2 out]
            n196 = Initialize Array(0, w299) -> (w298:i32[])
            n197 = property on="Listbox" class="LstBox (strict)"("Top Row"=w297, "Value"=w297, "Item Symbols"=w298) -> ()  [unwired: 2 in, 2 out]
          }
        }
      }
      event "Listbox": Key Down {
        # "Update symbols on the listbox\nLeft and right keys check and uncheck"
        n198 = event-data() -> ("VKey"=w303:T22)  [unwired: 1 in]
        n199 = case shown="\"Left\", \"Right\"" w303 {
          selector: w303 -> [w308 _]
          tunnel: eventvkey."Left" ("VKey") -> [w306 _]
          frame "Left", "Right" {
            n200 = Equal?(x=w306, y=w308) -> (x = y?=w307:bool)
            n201 = Select(t=0, s=w307, f=1) -> (s? t:f=w309:i32)
            n202 = property on="Listbox" class="LstBox (strict)"() -> ("Item Symbols"=w312:i32[])  [unwired: 2 in, 2 out]
            n203 = Replace Array Subset(array=w312, new element=w309, index="Listbox") -> (w311:i32[])
            n204 = property on="Listbox" class="LstBox (strict)"("Item Symbols"=w311) -> ()  [unwired: 2 in, 2 out]
          }
          frame Default {
          }
        }
      }
      event "DB Camera Config": Value Change {
        # "Show or hide the cluster of controls, store in ini file"
        n205 = event-data() -> ("NewVal"=w316:bool)  [unwired: 1 in]
        n206 = case shown="False" w316 {
          tunnel: w315 -> [w325 _]
          tunnel: [w318 w336] -> w314
          tunnel: w313 -> [w317 w336]
          frame False {
            w332 = "Camera"
            w335 = FALSE ("Visible")
            n207 = local read "Camera Settings"() -> (w324:T2)
            n208 = Index Array(array=w325) -> (element=w328:cluster{string[]})  [unwired: 1 in]
            n209 = Unbundle(w324) -> ("Frame Rate"=w323:i32, "Compression"=w322:i32, "Size"=w326:u16)
            n210 = Unbundle(w328) -> (w327:string[])
            n211 = Index Array(array=w327, index=w326) -> (element=w321:string)
            n212 = call-poly <vilib>:"Write Key.vi"("section"=w332, "value"=w321, "key"="Size", "refnum"=w317) -> ("refnum out"=w334:T20)  [unwired: 2 in, 5 out]
            n213 = call-poly <vilib>:"Write Key.vi"("section"=w332, "value"=w323, "key"="FrameRate", "refnum"=w334) -> ("refnum out"=w333:T20)  [unwired: 1 in, 6 out]
            n214 = property on="Camera Settings" class="Clust (strict)"("Visible"=w335) -> ()  [unwired: 2 in, 2 out]
            n215 = local write "DB Camera Config"(w335) -> ()
            n216 = call-poly <vilib>:"Write Key.vi"("section"=w332, "value"=w322, "key"="Compression", "refnum"=w333) -> ("refnum out"=w319:T20)  [unwired: 1 in, 6 out]
            n217 = call <vilib>:"Close Config Data.vi"("refnum"=w319) -> ("file path"=w320:path)  [unwired: 2 in, 8 out]
            n218 = call <vilib>:"Open Config Data.vi"("configuration file path"=w320) -> ("refnum"=w318:T20)  [unwired: 8 in, 2 out]
          }
          frame True {
            n219 = property on="Camera Settings" class="Clust (strict)"("Visible"=TRUE) -> ()  [unwired: 2 in, 2 out]
          }
        }
      }
      event "Camera Settings": Value Change {
        # "Update summary string when any elements of DB camera change"
        n220 = event-data() -> ("NewVal"=w349:T2)  [unwired: 1 in]
        n221 = Index Array(array=w345) -> (element=w344:cluster{string[]})  [unwired: 1 in]
        n222 = Unbundle(w349) -> ("Frame Rate"=w340:i32, "Compression"=w339:i32, "Size"=w342:u16)
        n223 = Unbundle(w344) -> (w343:string[])
        n224 = Index Array(array=w343, index=w342) -> (element=w341:string)
        n225 = Format Into String(format string="%s   %dfps   %d%%", w341, w340, w339) -> (resulting string=w346:string)  [unwired: 2 in, 1 out]
        n226 = Build Array(w346) -> (w347:string[])
        n227 = property on="DB Camera Config" class="Bool (strict)"("Strings [4]"=w347) -> ()  [unwired: 2 in, 2 out]
      }
      event "Motor.Enable": Value Change {
        # "When the test mode otor enable helper is set, update that\ntree row item's value"
        n228 = event-data() -> ("NewVal"=w355:bool)  [unwired: 1 in]
        n229 = Unbundle("Motor") -> ("Value"=w354:dbl)  [unwired: 1 out]
        n230 = Select(t=w354, s=w355, f=0.0) -> (s? t:f=w352:dbl)
        n231 = call <vilib>:"NT Write Number.vi"("Numeric"=w352, "Name"=w351) -> ()  [unwired: 9 in, 1 out]
      }
      event "Test Slider": Value Change {
        # "When the test mode slider helper is set, update that\ntree row item's value"
        n232 = event-data() -> ("NewVal"=w358:dbl)  [unwired: 1 in]
        n233 = call <vilib>:"NT Write Number.vi"("Numeric"=w358, "Name"=w359) -> ()  [unwired: 9 in, 1 out]
      }
      event "On/Off": Value Change {
        # "When the test mode on/off helper value is set, update that\ntree row item's value"
        n234 = event-data() -> ("NewVal"=w363:bool)  [unwired: 1 in]
        n235 = Boolean To (0,1)(Boolean=w363) -> (0, 1=w362:i16)
        n236 = call <vilib>:"NT Write Number.vi"("Numeric"=w362, "Name"=w361) -> ()  [unwired: 9 in, 1 out]
      }
      event "Rev/Fwd": Value Change {
        # "When the test mode helper value for relays is set, update that\ntree row item's value"
        n237 = event-data() -> ("NewVal.Forward"=w371:bool, "NewVal.Reverse"=w370:bool)  [unwired: 1 in]
        n238 = Boolean To (0,1)(Boolean=w371) -> (0, 1=w367:i16)
        n239 = Boolean To (0,1)(Boolean=w370) -> (0, 1=w369:i16)
        n240 = Negate(x=w369) -> (-x=w368:i16)
        n241 = Add(x=w367, y=w368) -> (x+y=w366:i16)
        n242 = call <vilib>:"NT Write Number.vi"("Numeric"=w366, "Name"=w365) -> ()  [unwired: 9 in, 1 out]
      }
      event "Test Ring": Value Change {
        # "When a test mode helper value is selected from the ring,\nset the tree item's variable to the string value"
        n243 = event-data() -> ("NewVal"=w375:u16)  [unwired: 1 in]
        n244 = property on="Test Ring" class="Ring (strict)"() -> ("Strings []"=w376:string[])  [unwired: 2 in, 2 out]
        n245 = Index Array(array=w376, index=w375) -> (element=w374:string)
        n246 = call <vilib>:"NT Write String.vi"("String"=w374, "Name"=w373) -> ()  [unwired: 9 in, 1 out]
      }
      event "Rec Mode": Value Change {
        # "Update globals for recording mode and path to read log from.\nClear when logging and let NetworkTables set path for vision to\nuse."
        n247 = event-data() -> ("NewVal"=w386:enum32{"Stop", "Record", "Playback"})  [unwired: 1 in]
        n248 = global write "WPI_DashboardLogging Global.vi" "Logging Filename"(path "") -> ()
        n249 = case shown="\"Playback\"" w386 {
          tunnel: w385 -> [_ w388 w396]
          tunnel: [_ _ w395] -> w382
          tunnel: [_ _ w394] -> _
          tunnel: w380 -> [_ _ w392]
          tunnel: cluster{i32, i32} {-250, 170} -> [_ _ w391]
          tunnel: [_ _ T23 {"Image Size"=TRUE, "Image Type"=TRUE, "Pixel Value"=TRUE, "ROI Information"=TRUE, "Zoom Factor"=FALSE} ("Image Information Shown:All Elements")] -> w378
          tunnel: [_ _ TRUE ("Zoom Factor")] -> w377
          frame Default {
          }
          frame "Stop", "Record" {
            # "Place Window too"
            n250 = invoke class="VI" method="FP.Close"(reference=w388) -> (reference out=w387:refnum<vi>)  [unwired: 2 in, 2 out]
            n251 = invoke class="VI" method="Abort VI"(reference=w387) -> ()  [unwired: 2 in, 3 out]
          }
          frame "Playback" {
            n252 = call "Open Playback Panel.vi"("Offset"=w391, "DB VI Ref"=w392, "Playback in"=w396) -> ("Playback out"=w393:refnum<vi>)  [unwired: 8 in]
            n253 = register-events(w393) -> (reference out=w395:refnum<event-registration>, error out=w394:errorcluster)  [unwired: 2 in]
          }
        }
        n254 = global write "WPI_DashboardLogging Global.vi" "Recording"(w386) -> ()
        n255 = property on="Camera Image" class="ImageControl"("Image Information Shown"=w378, "Image Information Visible"=w377) -> ()  [unwired: 2 in, 2 out]
        n256 = call <vilib>:"WPI_DashboardNT Log FieldName Cache.vi"("Operation"=enum16{"Lookup/Add", "Index", "Clear"}."Clear") -> ()  [unwired: 8 in, 3 out]
      }
      event Panel Close {
        w397 = enum32{"Stop", "Record", "Playback"}."Stop" ("Rec Mode")
        # "Playback window has been closed, abort"
        n257 = event-data() -> ()  [unwired: 1 in, 4 out]
        n258 = local write "Rec Mode"(w397) -> ()
        n259 = global write "WPI_DashboardLogging Global.vi" "Recording"(w397) -> ()
      }
      event Panel Close {
        # "Abort playback window and ourself"
        n260 = event-data() -> ()  [unwired: 1 in, 4 out]
        n261 = invoke class="VI" method="FP.Close"(reference=w402) -> (reference out=w401:refnum<vi>)  [unwired: 2 in, 2 out]
        n262 = invoke class="VI" method="Abort VI"(reference=w401) -> (error out=w400:errorcluster)  [unwired: 2 in, 2 out]
        n263 = invoke class="VI" method="Abort VI"(error in=w400) -> ()  [unwired: 2 in, 3 out]
      }
      event "Vision": Value Change {
        # "Enable/Disable Compression slider.\nHW USB is hard-coded into the camera"
        n264 = event-data() -> ("NewVal"=w408:u16)  [unwired: 1 in]
        n265 = Equal?(x=w408, y=u32 2 ("milliseconds to wait")) -> (x = y?=w406:bool)
        n266 = Select(t=T24."Disabled and Grayed Out" ("Disabled"), s=w406, f=T24."Enabled" ("Disabled")) -> (s? t:f=w403:T24)
        n267 = property on="Compression" class="Slide (strict)"("DisabledEnum"=w403) -> ()  [unwired: 2 in, 2 out]
      }
    }
  }
  n268 = while {
    tunnel: w38 -> [w411]
    i -> [w414]
    stop <- FALSE stop-if-true
    n269 = Wait (ms)(milliseconds to wait=u32 100) -> ()  [unwired: 1 out]
    n270 = case shown="\"Playback\"" "Rec Mode" {
      tunnel: w414 -> [_ _ w429]
      tunnel: [u32 2829099 ("Base Color") u32 11141120 ("Target Color") w418] -> w410
      frame "Stop", Default {
        # "Reset the color, extra updates don't cost much"
      }
      frame "Record" {
      }
      frame "Playback" {
        # "Playback"
        n271 = Quotient & Remainder(x=w429, y=u32 50 ("milliseconds to wait")) -> (x-y*floor(x/y)=w425:u32)  [unwired: 1 out]
        n272 = Divide(x=w425, y=u32 50 ("milliseconds to wait")) -> (x/y=w422:dbl)
        n273 = Multiply(x=6.283185307179586, y=w422) -> (x*y=w427:dbl)
        n274 = Sine(x=w427) -> (sin(x)=w426:dbl)
        n275 = Absolute Value(x=w426) -> (abs(x)=w419:dbl)
        n276 = call "Interpolate RGB Color.vi"("Proportion"=w419, "Target Color"=u32 30976, "Base Color"=u32 2829099) -> ("Result Color"=w418:u32)  [unwired: 8 in]
      }
    }
    n277 = property class="Pane"(reference=w411, "PaneColor"=w410) -> ()  [unwired: 1 in, 2 out]
  }
  n278 = TCP Create Listener(10:u16 1741 ("timeout ms (25000)")) -> (3:w1:refnum<k5>)  [unwired: 4 in, 2 out]
  n279 = while {
    tunnel: w1 -> [w431]
    stop <- FALSE stop-if-true
    n280 = TCP Wait On Listener(11:w431) -> (4:w430:refnum<k5>)  [unwired: 3 in, 4 out]
    n281 = local write "TCP"(w430) -> ()
  }
  n282 = property on="On/Off" class="Bool (strict)"("Visible"=w6) -> ()  [unwired: 2 in, 2 out]
  n283 = property on="Motor" class="Clust (strict)"("Visible"=w6) -> ()  [unwired: 2 in, 2 out]
  n284 = property on="Progress" class="Clust (strict)"("Visible"=w6) -> ()  [unwired: 2 in, 2 out]
  n285 = property on="Test Ring" class="Ring (strict)"("Visible"=w6) -> ()  [unwired: 2 in, 2 out]
  n286 = property on="Rev/Fwd" class="Clust (strict)"("Visible"=w6) -> ()  [unwired: 2 in, 2 out]
  n287 = property on="Camera Settings" class="Clust (strict)"("Visible"=w6) -> ()  [unwired: 2 in, 2 out]
  n288 = local write "DB Camera Config"(w6) -> ()
  n289 = global write "WPI_DashboardLogging Global.vi" "Recording"(w32) -> ()
  n290 = local write "Rec Mode"(w32) -> ()
